vi "Keep MagField.vi"(8 "Actual_Current":dbl, 10 "Desired_M_Field 2":dbl, 11 "Actual_M_Field":dbl) -> (2 "Objetive current":dbl)   [LabVIEW 2017]
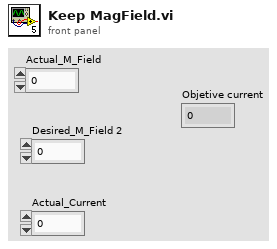
[diagram p1: front panel]
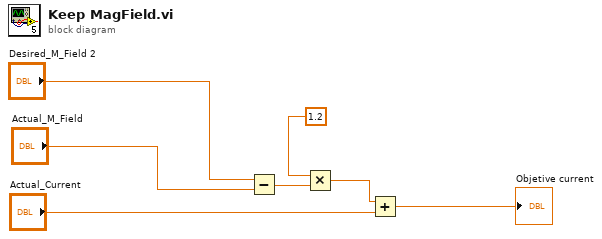
[diagram p0: block diagram]
diagram:
  n1 = Subtract(x="Desired_M_Field 2", y="Actual_M_Field") -> (x-y=w5:dbl)
  n2 = Multiply(x=1.2, y=w5) -> (x*y=w2:dbl)
  n3 = Add(x=w2, y="Actual_Current") -> (x+y=→"Objetive current":dbl)
